vi "Play Path.vi"(4 "Align for Path":bool, 5 "Right Setpoint (Turning)":dbl, 6 "Synchronication":enum16{"Start", "Wait"}(ring), 7 "Description":string, 8 "Command Info In":T1, 9 "Reverse (T) / Normal (F)":bool, 10 "Path Reversed":bool, 11 "Path":path) -> (0 "Command Info Out":T1)   [LabVIEW 2019]
doc: "This VI notifies the subsystem to the new setpoint."
uses:
  <vilib>/Rock Robotics/WPI/Framework/Command Status Info.ctl
  <vilib>/Rock Robotics/WPI/Framework/Completion Status.ctl
  <vilib>/Rock Robotics/WPI/Framework/Completion Notifier.ctl
  2020 Robot/Drive/Implementation/Drive Setpoints.ctl
  2020 Robot/Drive/Implementation/Drive Operations.ctl
  Bordeaux/Command Stuff/Single Cmd Info.ctl
  <vilib>/picture/picture.llb/imagedata.ctl
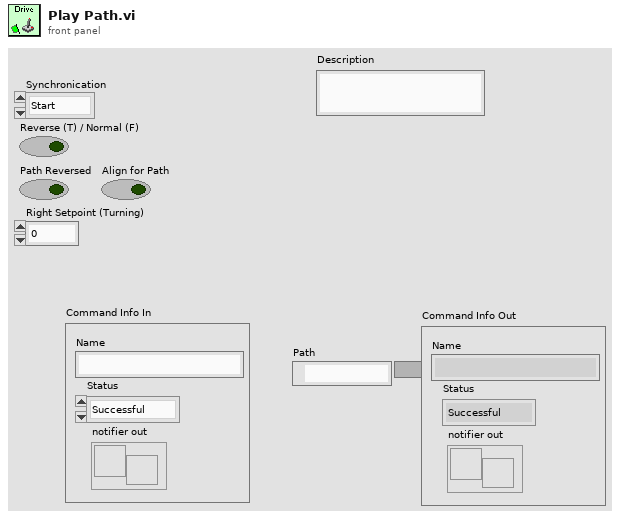
[diagram p1: front panel]
types:
  T1 = typedef "Command Status Info.ctl" = cluster{"Name":string, "Status":T2, "notifier out":T3}
  T2 = typedef "Completion Status.ctl" = enum16{"Successful", "Aborted", "Incomplete"}
  T3 = typedef "Completion Notifier.ctl" = refnum<notifier>
  T4 = cluster{"V":dbl[], "Theta":dbl[], "Sample Period":dbl}
  T5 = typedef "Drive Operations.ctl" = enum16{"Reserve", "Read Current", "Immediate", "Pod Racer", "Ball AA", "Feeder Station AA", "Play Back From Log"}
  T6 = typedef "Drive Setpoints.ctl" = cluster{"Operation":T5, "Forwards/Backwards":dbl, "Turning":dbl, "Transmition Engaged?":bool, "Reverse (T) / Normal (F)":bool, "Field Align?":bool, "Auto Path Data":cluster{"V":dbl[], "Theta":dbl[], "Sample Period":dbl}, "Path Reversed":bool, "Commands":cluster{"Time (s)":dbl, T7, bool}[]}
  T7 = typedef "Single Cmd Info.ctl" = cluster{"Name":string, "CPTM.DataType":variant, "All Control Values Variant":cluster{"Name":string, "Variant Data":variant}[], "icon full":T8, "icon scaled":T8, "Path":path, "Subsystem Color":u32}
  T8 = typedef "imagedata.ctl" = cluster{"image type":i32, "image depth":i32, "image":u8[], "mask":u8[], "colors":u32[], "Rectangle":cluster{"left":i16, "top":i16, "right":i16, "bottom":i16}}
  T9 = cluster{"Segment Name":string, "Type":enum16{"Accel Straight", "Const Straight", "Blend", "Circle"}, "Traj Pos Points":cluster{"x":dbl, "y":dbl, "th":dbl}[], "Traj Vel Points":cluster{"V":dbl, "th":dbl}[], "Accel Index":i32, "Decel Index":i32}[]
  T10 = cluster{"Path Backwards":bool, "Robot Backwards":bool}
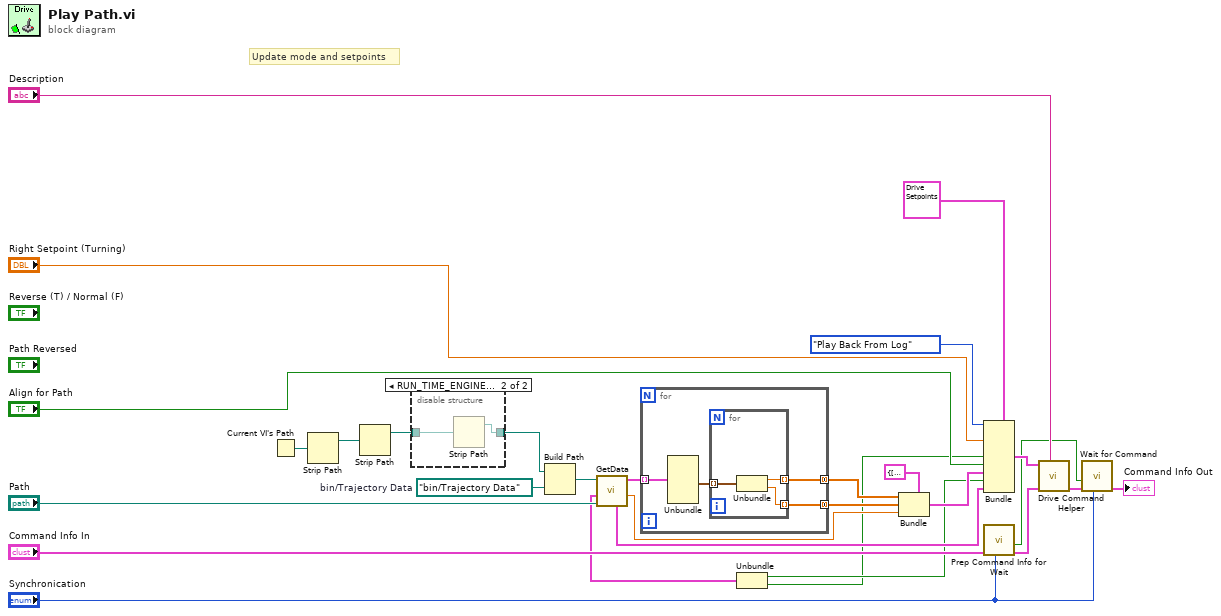
[diagram p0: block diagram]
diagram:
  w14 = path "bin/Trajectory Data"  # bin/Trajectory Data
  # "Update mode and setpoints"
  n1 = Current VI's Path() -> (path=w16:path)
  n2 = Strip Path(path=w16) -> (stripped path=w15:path)  [unwired: 1 out]
  n3 = Strip Path(path=w15) -> (stripped path=w12:path)  [unwired: 1 out]
  n4 = disable-structure shown="RUN_TIME_ENGINE==True, Default" {
    disable-tunnel: [w30 w31] -> w13
    disable-tunnel: w12 -> [w30 w32]
    frame condition #0 (active) {
    }
    frame condition #1 {
      n5 = Strip Path(path=w32) -> (stripped path=w31:path)  [unwired: 1 out]
    }
  }
  n6 = Build Path(base path=w13, name or relative path=w14) -> (appended path=w17:path)
  n7 = call "GetData.vi"("File"="Path", "file (use dialog)"=w17) -> ("Sample Period (s)"=w6:dbl, "Trajectory Data"=w18:T9, "Commands"=w4:cluster{"Time (s)":dbl, T7, bool}[], "Cluster 2"=w3:T10)  [unwired: 1 in, 5 out]
  n8 = for {
    tunnel: [w36] -> w11 mode=concatenating
    tunnel: [w35] -> w10 mode=concatenating
    tunnel: w18 -> [w33] mode=indexing
    n9 = Unbundle(w33) -> ("Traj Vel Points"=w34:cluster{"V":dbl, "th":dbl}[])  [unwired: 5 out]
    n10 = for {
      tunnel: w34 -> [w37] mode=indexing
      tunnel: [w39] -> w36 mode=indexing
      tunnel: [w38] -> w35 mode=indexing
      n11 = Unbundle(w37) -> ("V"=w39:dbl, "th"=w38:dbl)
    }
  }
  n12 = Unbundle(w3) -> ("Path Backwards"=w2:bool, "Robot Backwards"=w1:bool)
  n13 = Bundle(cluster=T4 {"V"=[], "Theta"=[], "Sample Period"=0.0} ("Auto Path Data"), "V"=w11, "Theta"=w10, "Sample Period"=w6) -> (w5:T4)
  n14 = Bundle(cluster=T6 {"Operation"=enum."Immediate", "Forwards/Backwards"=0.0, "Turning"=0.0, "Transmition Engaged?"=FALSE, "Reverse (T) / Normal (F)"=FALSE, "Field Align?"=FALSE, "Auto Path Data"={"V"=[], "Theta"=[], "Sample Period"=0.0}, "Path Reversed"=FALSE, "Commands"=[]} ("SubSystem Data"), "Operation"=Drive_Operations."Play Back From Log", "Turning"="Right Setpoint (Turning)", "Reverse (T) / Normal (F)"=w1, "Field Align?"="Align for Path", "Auto Path Data"=w5, "Path Reversed"=w2, "Commands"=w4) -> (w27:T6)  [unwired: 2 in]
  n15 = call <vilib>:"Prep Command Info for Wait.vi"("Synchronication"="Synchronication", "Command Info"="Command Info In") -> ("Command Info"=w25:T1, "Allocated"=w21:bool)  [unwired: 8 in]
  n16 = call "Drive Command Helper.vi"("Description"="Description", "Command Info In"=w25, "SubSystem Data"=w27) -> ("Command Info Out"=w24:T1)  [unwired: 6 in, 2 out]
  n17 = call <vilib>:"Wait for Command.vi"("Synchronication"="Synchronication", "Command Info in"=w24, "Allocated"=w21) -> ("Command Info out"=→"Command Info Out":T1)  [unwired: 8 in]
